vi "Configure Stream UE9.vi"(1 "Stream Timeout":dbl=1500.0 format="%.2f", 4 "External Scan Trigger":bool, 5 "Scan Clock Output":bool, 6 "Wait Mode":string="LJ_swNONE", 7 "PC buffer size (seconds)":dbl=5.0 format="%.2f", 8 "error in":errorcluster, 9 "Scan List":u8[](array[numeric])=[0, 1, 2, 3], 10 "Scan Rate (Hz)":dbl=1000.0 format="%.2f", 11 "Handle In":i32) -> (0 "error out":errorcluster, 2 "PC buffer size (samples)":i32=5, 3 "Handle Out":i32)   [LabVIEW 2020]
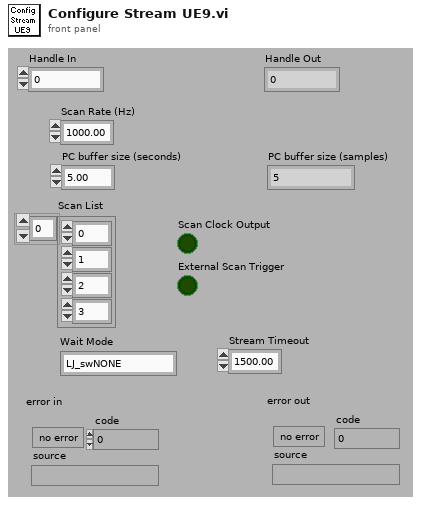
[diagram p1: front panel]
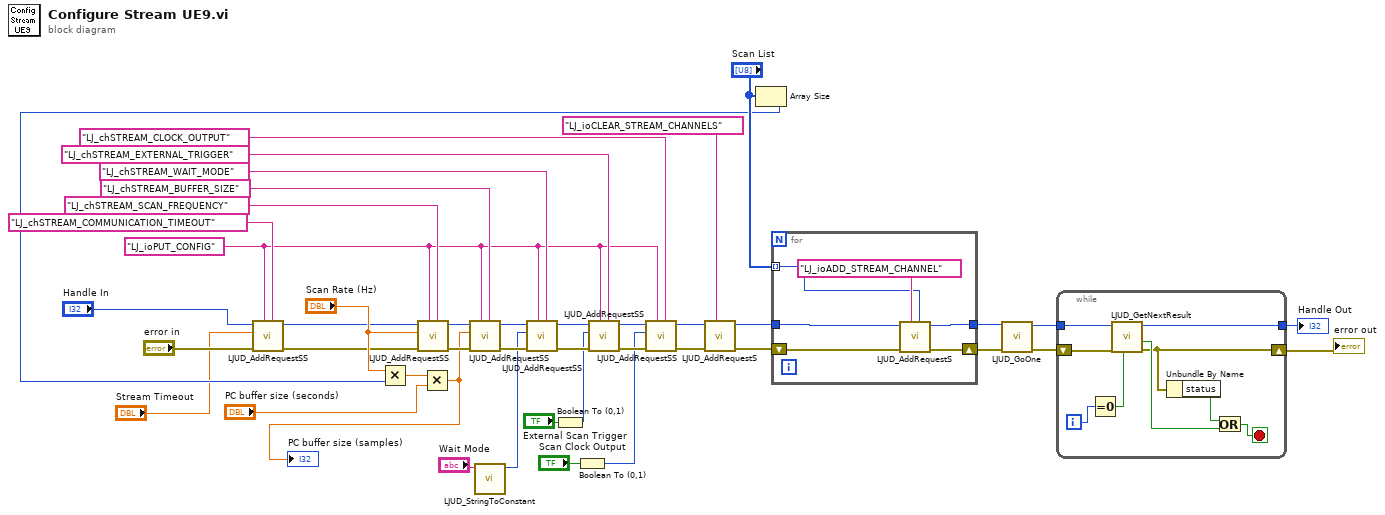
[diagram p0: block diagram]
diagram:
  w6 = "LJ_ioPUT_CONFIG" ("IOType")
  n1 = call "LJUD_AddRequestSS.vi"("Channel"="LJ_chSTREAM_COMMUNICATION_TIMEOUT" ("IOType"), "IOType"=w6, "error in"="error in", "Value"="Stream Timeout", "Handle In"="Handle In") -> ("error out"=w2:errorcluster, "Handle Out"=w4:i32)  [unwired: 5 in]
  n2 = call "LJUD_AddRequestSS.vi"("Channel"="LJ_chSTREAM_SCAN_FREQUENCY" ("IOType"), "IOType"=w6, "error in"=w2, "Value"="Scan Rate (Hz)", "Handle In"=w4) -> ("error out"=w41:errorcluster, "Handle Out"=w43:i32)  [unwired: 5 in]
  n3 = call "LJUD_StringToConstant.vi"("String"="Wait Mode") -> ("Constant Number"=w11:i32)  [unwired: 9 in, 1 out]
  n4 = Boolean To (0,1)(Boolean="External Scan Trigger") -> (0, 1=w16:i16)
  n5 = Boolean To (0,1)(Boolean="Scan Clock Output") -> (0, 1=w13:i16)
  n6 = Array Size(array="Scan List") -> (size(s)=w26:i32)
  n7 = Multiply(x="Scan Rate (Hz)", y=w26) -> (x*y=w31:dbl)
  n8 = Multiply(x=w31, y="PC buffer size (seconds)") -> (x*y=w8:dbl)
  "PC buffer size (samples)" <- w8
  n9 = call "LJUD_AddRequestSS.vi"("Channel"="LJ_chSTREAM_BUFFER_SIZE" ("IOType"), "IOType"=w6, "error in"=w41, "Value"=w8, "Handle In"=w43) -> ("error out"=w40:errorcluster, "Handle Out"=w42:i32)  [unwired: 5 in]
  n10 = call "LJUD_AddRequestSS.vi"("Channel"="LJ_chSTREAM_WAIT_MODE" ("IOType"), "IOType"=w6, "error in"=w40, "Value"=w11, "Handle In"=w42) -> ("error out"=w21:errorcluster, "Handle Out"=w22:i32)  [unwired: 5 in]
  n11 = call "LJUD_AddRequestSS.vi"("Channel"="LJ_chSTREAM_EXTERNAL_TRIGGER" ("IOType"), "IOType"=w6, "error in"=w21, "Value"=w16, "Handle In"=w22) -> ("error out"=w24:errorcluster, "Handle Out"=w23:i32)  [unwired: 5 in]
  n12 = call "LJUD_AddRequestSS.vi"("Channel"="LJ_chSTREAM_CLOCK_OUTPUT" ("IOType"), "IOType"=w6, "error in"=w24, "Value"=w13, "Handle In"=w23) -> ("error out"=w17:errorcluster, "Handle Out"=w18:i32)  [unwired: 5 in]
  n13 = call "LJUD_AddRequestS.vi"("IOType"="LJ_ioCLEAR_STREAM_CHANNELS", "error in"=w17, "Handle In"=w18) -> ("error out"=w29:errorcluster, "Handle Out"=w30:i32)  [unwired: 7 in]
  n14 = for {
    tunnel: w30 -> [w49]
    shift-right: [w46] -> w35
    shift-left: w29 -> [w47]
    tunnel: "Scan List" -> [w44] mode=indexing
    tunnel: [w45] -> w36
    n15 = call "LJUD_AddRequestS.vi"("Channel"=w44, "IOType"="LJ_ioADD_STREAM_CHANNEL", "error in"=w47, "Handle In"=w49) -> ("error out"=w46:errorcluster, "Handle Out"=w45:i32)  [unwired: 6 in]
  }
  n16 = call "LJUD_GoOne.vi"("error in"=w35, "Handle In"=w36) -> ("error out"=w10:errorcluster, "Handle Out"=w33:i32)  [unwired: 8 in]
  n17 = while {
    shift-left: w10 -> [w51]
    shift-right: [w50] -> w9
    tunnel: [w54] -> w34
    tunnel: w33 -> [w56]
    i -> [w53]
    stop <- w58 stop-if-true
    n18 = Equal To 0?(x=w53) -> (x = 0?=w57:bool)
    n19 = call "LJUD_GetNextResult.vi"("GetFirst"=w57, "error in"=w51, "Handle In"=w56) -> ("error out"=w50:errorcluster, "LJE_NO_MORE_DATA_AVAILABLE"=w52:bool, "Handle Out"=w54:i32)  [unwired: 3 in, 3 out]
    n20 = Unbundle By Name(w50) -> ("status"=w55:bool)
    n21 = Or(x=w55, y=w52) -> (x .or. y?=w58:bool)
  }
  "Handle Out" <- w34
  "error out" <- w9
